vi "Last Ack Creator Queue.vi"(10 "Queue":refnum<class "Queue.lvclass">, 11 "Base Event in":refnum<class "Base Event.lvclass">) -> (3 "Base Event out":refnum<class "Base Event.lvclass">)   [LabVIEW 2021, in "jettl.lvlib" / "Base Event.lvlib" / "Base Event.lvclass"]
uses:
  Base Event.lvclass
  Queue/Queue.lvclass
  Base Event.lvclass/Base Event.ctl
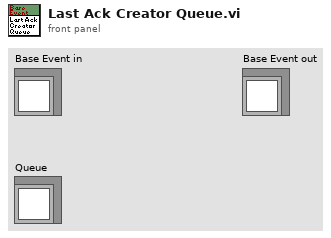
[diagram p1: front panel]
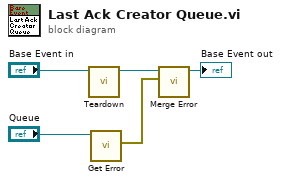
[diagram p0: block diagram]
diagram:
  n1 = call-dynamic "Teardown.vi"("Base Event in"="Base Event in") -> ("Base Event out"=w1:refnum<class "Base Event.lvclass">)  [unwired: 10 in]
  n2 = call-dynamic "Get Error.vi"("jettl in"="Queue") -> ("Error"=w3:errorcluster)  [unwired: 10 in]
  n3 = call-dynamic "Merge Error.vi"("Error"=w3, "Base Event in"=w1) -> ("Base Event out"=→"Base Event out":refnum<class "Base Event.lvclass">)  [unwired: 9 in]
